vi "Reinit_Default.vi"(8 "error in (no error)":errorcluster, 9 "System data in":T1, 10 "Wash Options":refnum<vi>, 11 "VI in":refnum<vi>) -> (0 "error out":errorcluster, 3 "System data out":T1)   [LabVIEW 2023]
uses:
  Controls/System_Data.ctl
  Controls/Wash Options.ctl
  Controls/State.ctl
  a808926f-1dd4-47a3-9706-949a4a91f160.vi
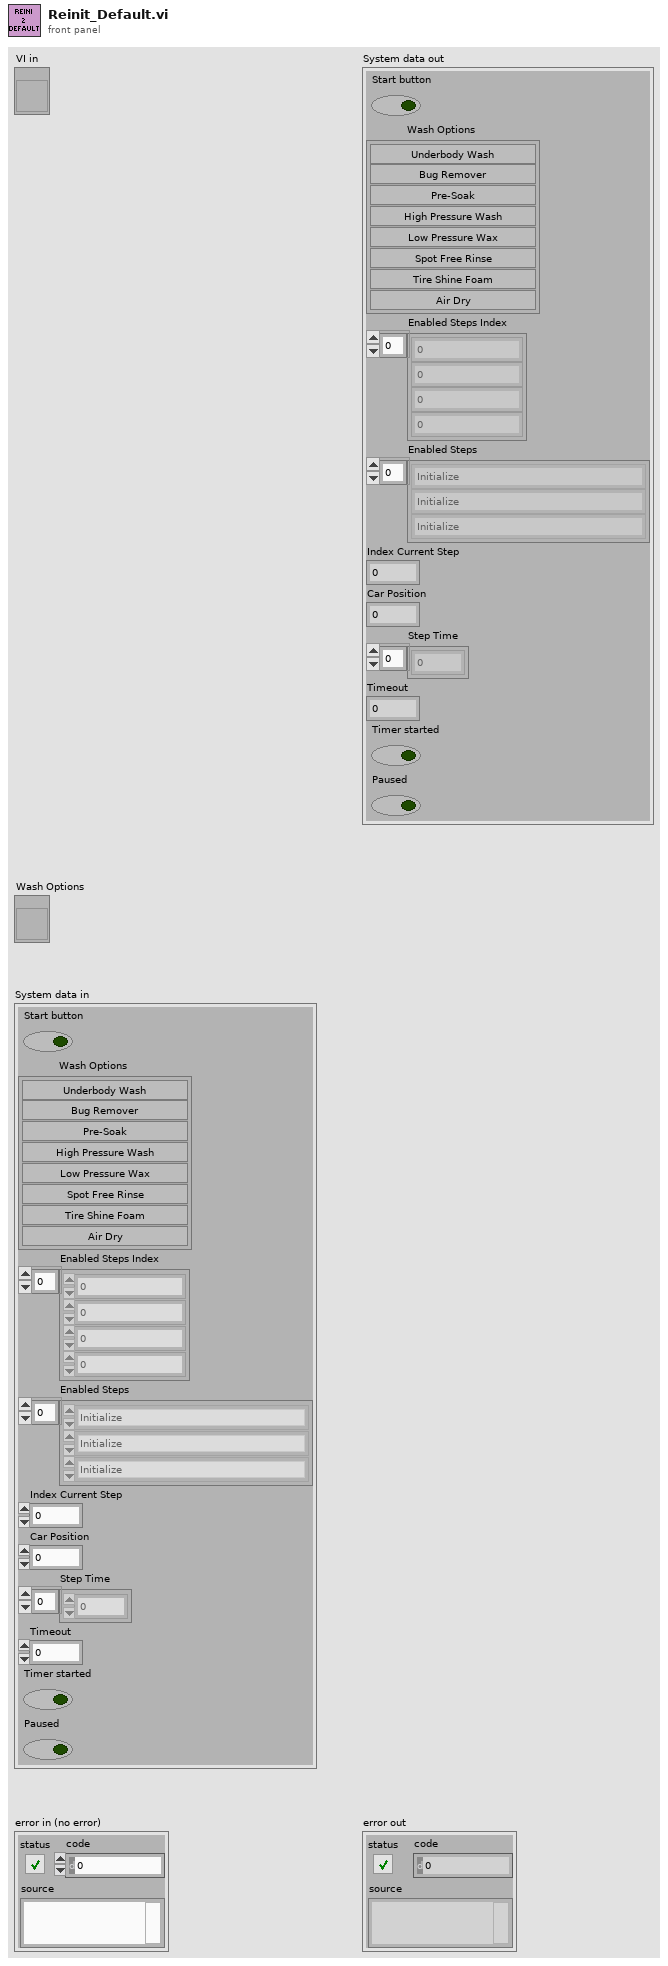
[diagram p1: front panel]
types:
  T1 = typedef "System_Data.ctl" = cluster{"Start button":bool, "Wash Options":T2, "Enabled Steps Index":i32[], "Enabled Steps ":T3[], "Index Current Step":i32, "Car Position":u8, "Step Time":dbl[], "Timeout":i32, "Timer started":bool, "Paused":bool}
  T2 = typedef "Wash Options.ctl" = cluster{"Underbody Wash":bool, "Bug Remover":bool, "Pre-Soak":bool, "High Pressure Wash":bool, "Low Pressure Wax":bool, "Spot Free Rinse":bool, "Tire Shine Foam":bool, "Air Dry":bool}
  T3 = typedef "State.ctl" = enum16{"Initialize", "Wait for Something", "Step Completed", "Save Wash Options", "Start Process", "Car Position", "Order Steps to follow", "Underbody Wash", "Bug Remover", "Pre-Soak", "High Pressure Wash", "Low Pressure Wax", "Spot Free Rinse", "Tire Shine Foam", "Air Dry", "Vehicle out of position", "Exit", "Process Complete", "Stop Application"}
  T4 = enum8{"Enabled", "Disabled", "Disabled and Grayed Out"}
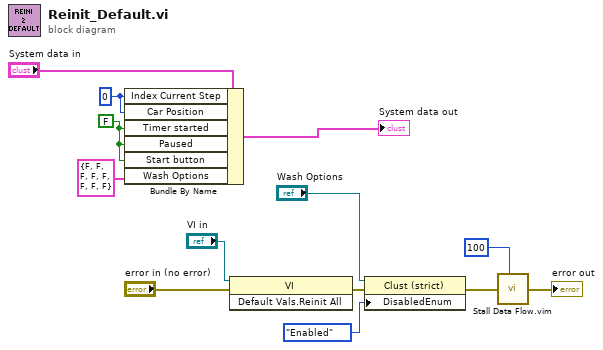
[diagram p0: block diagram]
diagram:
  w3 = FALSE
  w12 = 0 ("Index Current Step")
  n1 = Bundle By Name(cluster="System data in", "Index Current Step"=w12, "Car Position"=w12, "Timer started"=w3, "Paused"=w3, "Start button"=w3, "Wash Options"=T2 {"Underbody Wash"=FALSE, "Bug Remover"=FALSE, "Pre-Soak"=FALSE, "High Pressure Wash"=FALSE, "Low Pressure Wax"=FALSE, "Spot Free Rinse"=FALSE, "Tire Shine Foam"=FALSE, "Air Dry"=FALSE}) -> (→"System data out":T1)
  n2 = invoke class="VI" method="Default Vals.Reinit All"(reference="VI in", error in="error in (no error)") -> (error out=w13:errorcluster)  [unwired: 1 in, 2 out]
  n3 = property class="Clust (strict)"(reference="Wash Options", error in=w13, "DisabledEnum"=T4."Enabled" ("Disabled")) -> (error out=w9:errorcluster)  [unwired: 1 out]
  n4 = call "Stall Data Flow.vim"("value in"=w9, "milliseconds to wait"=u32 100) -> ("value out"=→"error out":errorcluster)  [unwired: 1 out]
